vi "InitaliseODrive.vi"(8 "error in (no error)":errorcluster, 11 "FPGA Interface in":refnum<k20>) -> (0 "error out":errorcluster, 1 "Encoder Index Position":i16, 3 "FPGA Interface out":refnum<k20>)   [LabVIEW 2016]
uses:
  <vilib>/Utility/error.llb/Error Cluster From Error Code.vi
  <vilib>/rvi/errors/niLvFpgaAdjustHostInterfaceError.vi
  <vilib>/RVI Host/nirviSupport.llb/nirviErrorClusterFromErrorCode.vi
  <vilib>/rvi/interface/nirviMethod/nirviMethod.xnode
  <vilib>/rvi/interface/nirviReadWriteControl/nirviReadWriteControl.xnode
  NiFpgaLv.dll
  <vilib>/rvi/interface/Simulation/niFpgaSimulationCallBeginRW.vi
  <vilib>/rvi/errors/niLvFpgaMergeErrorWithErrorCode.vi
  <vilib>/FPGAPlugInAG/Dynamic/niLvFpga_WriteFifo_Dynamic.vi
  <vilib>/rvi/interface/nirviMethod/StockFPGA_InlinedMethodWaitForSingleIRQ.vi
  <vilib>/FPGAPlugInAG/Dynamic/niLvFpga_WaitOnIrq_Dynamic.vi
  <vilib>/FPGAPlugInAG/Dynamic/niLvFpga_AcknowledgeIrq_Dynamic.vi
  <vilib>/FPGAPlugInAG/Dynamic/niLvFpga_StartFifo_Dynamic.vi
panel:
  out "Velocity Axis0":i16
  out "ODrive State":u8
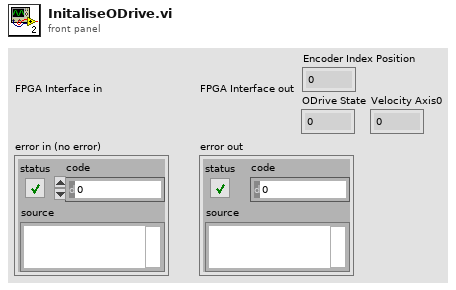
[diagram p1: front panel]
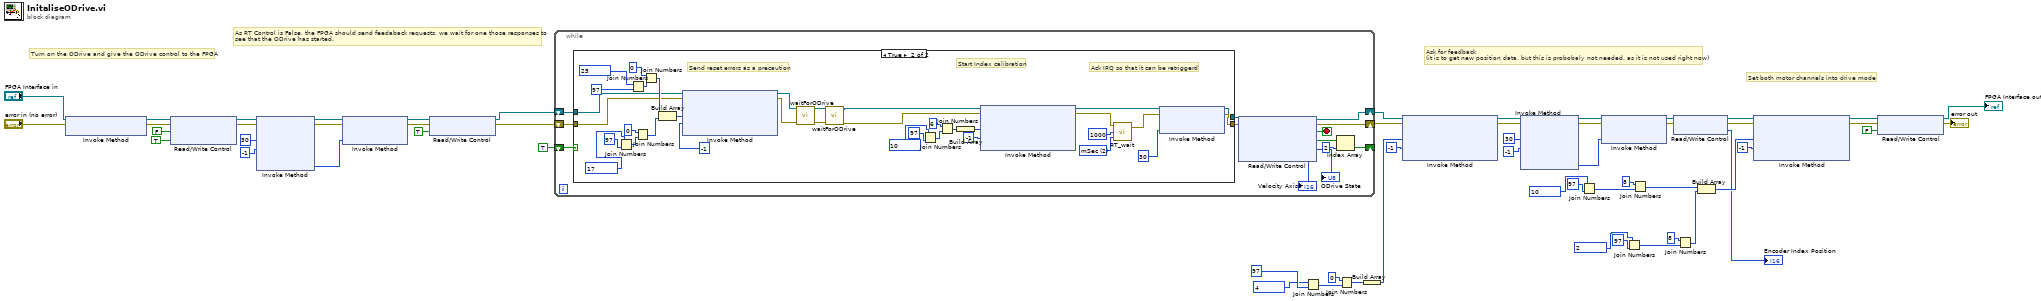
[diagram p0: block diagram]
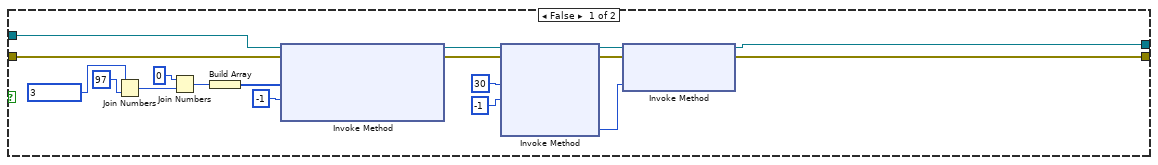
[diagram p2: hidden frame]
diagram:
  # "Set both motor channels into drive mode"
  # "Ask for feedback\n(it is to get new position data, but this is probobaly not needed, as it is not used right now)"
  # "Turn on the ODrive and give the ODrive control to the FPGA"
  # "As RT Control is False, the FPGA should send feedaback requests, we wait for one those responses to\nsee that the ODrive has started."
  n1 = xnode "Invoke Method"("FPGA VI Reference In"="FPGA Interface in", "error in"="error in (no error)") -> ("FPGA VI Reference Out"=w51:refnum<k20>, "error out"=w52:errorcluster)
  n2 = xnode "Read/Write Control"("FPGA VI Reference In"=w51, "error in"=w52, "ODrive RT Control"=FALSE, "MotorsON"=TRUE) -> ("FPGA VI Reference Out"=w27:refnum<k20>, "error out"=w26:errorcluster)
  n3 = xnode "Invoke Method"("FPGA VI Reference In"=w27, "error in"=w26, "IRQ Number(s)"=30, "Timeout (ms)"=-1) -> ("FPGA VI Reference Out"=w32:refnum<k20>, "error out"=w29:errorcluster, "IRQ(s) Asserted"=w30:i32)  [unwired: 1 out]
  n4 = xnode "Invoke Method"("FPGA VI Reference In"=w32, "error in"=w29, "IRQ Number(s)"=w30) -> ("FPGA VI Reference Out"=w24:refnum<k20>, "error out"=w25:errorcluster)
  n5 = xnode "Read/Write Control"("FPGA VI Reference In"=w24, "error in"=w25, "ODrive RT Control"=TRUE) -> ("FPGA VI Reference Out"=w10:refnum<k20>, "error out"=w11:errorcluster)
  n6 = while {
    shift-right: [w70] -> w44
    shift-left: w11 -> [w67]
    shift-right: [w69] -> w43
    shift-left: w10 -> [w66]
    shift-right: [w65] -> _
    shift-left: TRUE -> [w62]
    stop <- w68 stop-if-true
    n7 = case shown="True" w62 {
      tunnel: w67 -> [w83 w113]
      tunnel: w66 -> [w82 w112]
      tunnel: [w74 w109] -> w60
      tunnel: [w73 w108] -> w61
      frame False {
        n8 = Join Numbers(hi=u8 3 ("lo"), lo=u8 97) -> ((hi.lo)=w88:u16)
        n9 = Join Numbers(hi=u16 0, lo=w88) -> ((hi.lo)=w86:u32)
        n10 = Build Array(w86) -> (w85:u32[])
        n11 = xnode "Invoke Method"("FPGA VI Reference In"=w82, "error in"=w83, "Data"=w85, "Timeout (ms)"=-1) -> ("FPGA VI Reference Out"=w75:refnum<k20>, "error out"=w76:errorcluster)  [unwired: 1 out]
        n12 = xnode "Invoke Method"("FPGA VI Reference In"=w75, "error in"=w76, "IRQ Number(s)"=30, "Timeout (ms)"=-1) -> ("FPGA VI Reference Out"=w78:refnum<k20>, "error out"=w80:errorcluster, "IRQ(s) Asserted"=w79:i32)  [unwired: 1 out]
        n13 = xnode "Invoke Method"("FPGA VI Reference In"=w78, "error in"=w80, "IRQ Number(s)"=w79) -> ("FPGA VI Reference Out"=w73:refnum<k20>, "error out"=w74:errorcluster)
      }
      frame True {
        w106 = u16 2 items=["Ticks", "uSec", "mSec"] ("Counter Units")
        # "Ack IRQ so that it can be retriggerd"
        # "Start Index calibration"
        # "Send reset errors as a precaution"
        n14 = Join Numbers(hi=u8 17 ("lo"), lo=u8 97) -> ((hi.lo)=w95:u16)
        n15 = Join Numbers(hi=u8 25 ("lo"), lo=u8 97) -> ((hi.lo)=w118:u16)
        n16 = Join Numbers(hi=u16 0, lo=w95) -> ((hi.lo)=w93:u32)
        n17 = Join Numbers(hi=u16 0, lo=w118) -> ((hi.lo)=w116:u32)
        n18 = Build Array(w116, w93) -> (w115:u32[])
        n19 = xnode "Invoke Method"("FPGA VI Reference In"=w112, "error in"=w113, "Data"=w115, "Timeout (ms)"=-1) -> ("FPGA VI Reference Out"=w110:refnum<k20>, "error out"=w111:errorcluster)  [unwired: 1 out]
        n20 = call "waitForODrive.vi"("error in (no error)"=w111, "Refnum in"=w110) -> ("error out"=w92:errorcluster, "Refnum out"=w91:refnum<k20>)  [unwired: 8 in]
        n21 = call "waitForODrive.vi"("error in (no error)"=w92, "Refnum in"=w91) -> ("error out"=w90:errorcluster, "Refnum out"=w89:refnum<k20>)  [unwired: 8 in]
        n22 = Join Numbers(hi=u8 10 ("lo"), lo=u8 97) -> ((hi.lo)=w123:u16)
        n23 = Join Numbers(hi=u16 6, lo=w123) -> ((hi.lo)=w121:u32)
        n24 = Build Array(w121) -> (w120:u32[])
        n25 = xnode "Invoke Method"("FPGA VI Reference In"=w89, "error in"=w90, "Data"=w120, "Timeout (ms)"=-1) -> ("FPGA VI Reference Out"=w102:refnum<k20>, "error out"=w104:errorcluster)  [unwired: 1 out]
        n26 = call "RT_wait.vi"("Counter Units"=w106, "Count(mSec)"=u32 1000, "error in (no error)"=w104) -> ("error out"=w103:errorcluster)  [unwired: 1 in, 1 out]
        n27 = xnode "Invoke Method"("FPGA VI Reference In"=w102, "error in"=w103, "IRQ Number(s)"=30) -> ("FPGA VI Reference Out"=w108:refnum<k20>, "error out"=w109:errorcluster)
      }
    }
    n28 = xnode "Read/Write Control"("FPGA VI Reference In"=w61, "error in"=w60) -> ("FPGA VI Reference Out"=w69:refnum<k20>, "error out"=w70:errorcluster, "ODrive Encoder ready"=w68:bool, "ODrive Error Flags"=w64:bool[], "ODrive State"=→"ODrive State":u8, "Velocity Axis0"=→"Velocity Axis0":i16)
    n29 = Index Array(array=w64, index=2) -> (element=w65:bool)
  }
  n30 = Join Numbers(hi=u8 4 ("lo"), lo=u8 97) -> ((hi.lo)=w48:u16)
  n31 = Join Numbers(hi=u16 0, lo=w48) -> ((hi.lo)=w46:u32)
  n32 = Build Array(w46) -> (w45:u32[])
  n33 = xnode "Invoke Method"("FPGA VI Reference In"=w43, "error in"=w44, "Data"=w45, "Timeout (ms)"=-1) -> ("FPGA VI Reference Out"=w36:refnum<k20>, "error out"=w37:errorcluster)  [unwired: 1 out]
  n34 = xnode "Invoke Method"("FPGA VI Reference In"=w36, "error in"=w37, "IRQ Number(s)"=30, "Timeout (ms)"=-1) -> ("FPGA VI Reference Out"=w41:refnum<k20>, "error out"=w38:errorcluster, "IRQ(s) Asserted"=w39:i32)  [unwired: 1 out]
  n35 = Join Numbers(hi=u8 10 ("lo"), lo=u8 97) -> ((hi.lo)=w20:u16)
  n36 = xnode "Invoke Method"("FPGA VI Reference In"=w41, "error in"=w38, "IRQ Number(s)"=w39) -> ("FPGA VI Reference Out"=w34:refnum<k20>, "error out"=w35:errorcluster)
  n37 = Join Numbers(hi=u8 2 ("lo"), lo=u8 97) -> ((hi.lo)=w4:u16)
  n38 = Join Numbers(hi=u16 8, lo=w20) -> ((hi.lo)=w22:u32)
  n39 = xnode "Read/Write Control"("FPGA VI Reference In"=w34, "error in"=w35) -> ("FPGA VI Reference Out"=w19:refnum<k20>, "error out"=w18:errorcluster, "Position Axis1"=→"Encoder Index Position":i16)
  n40 = Join Numbers(hi=u16 8, lo=w4) -> ((hi.lo)=w1:u32)
  n41 = Build Array(w22, w1) -> (w23:u32[])
  n42 = xnode "Invoke Method"("FPGA VI Reference In"=w19, "error in"=w18, "Data"=w23, "Timeout (ms)"=-1) -> ("FPGA VI Reference Out"=w17:refnum<k20>, "error out"=w16:errorcluster)  [unwired: 1 out]
  n43 = xnode "Read/Write Control"("FPGA VI Reference In"=w17, "error in"=w16, "ODrive RT Control"=FALSE) -> ("FPGA VI Reference Out"=→"FPGA Interface out":refnum<k20>, "error out"=→"error out":errorcluster)
